vi "ContCompilePreSeq.vi"(11 "Compiler Settings In":T3={"Python Path"=path "", "Main File"="", "Meta File"="", "Aux File"="makesequence.py", "Pre File"="metascript.txt"}) -> (3 "Pre Pulse Seq":T1)   [LabVIEW 2019]
uses:
  PulseCompiler/CompilerSettings.ctl
  PulseControl.ctl
  Compiler/Params.ctl
panel:
  out "error out 2":errorcluster
  in  "Stepnum":i32
  out "standard error":string
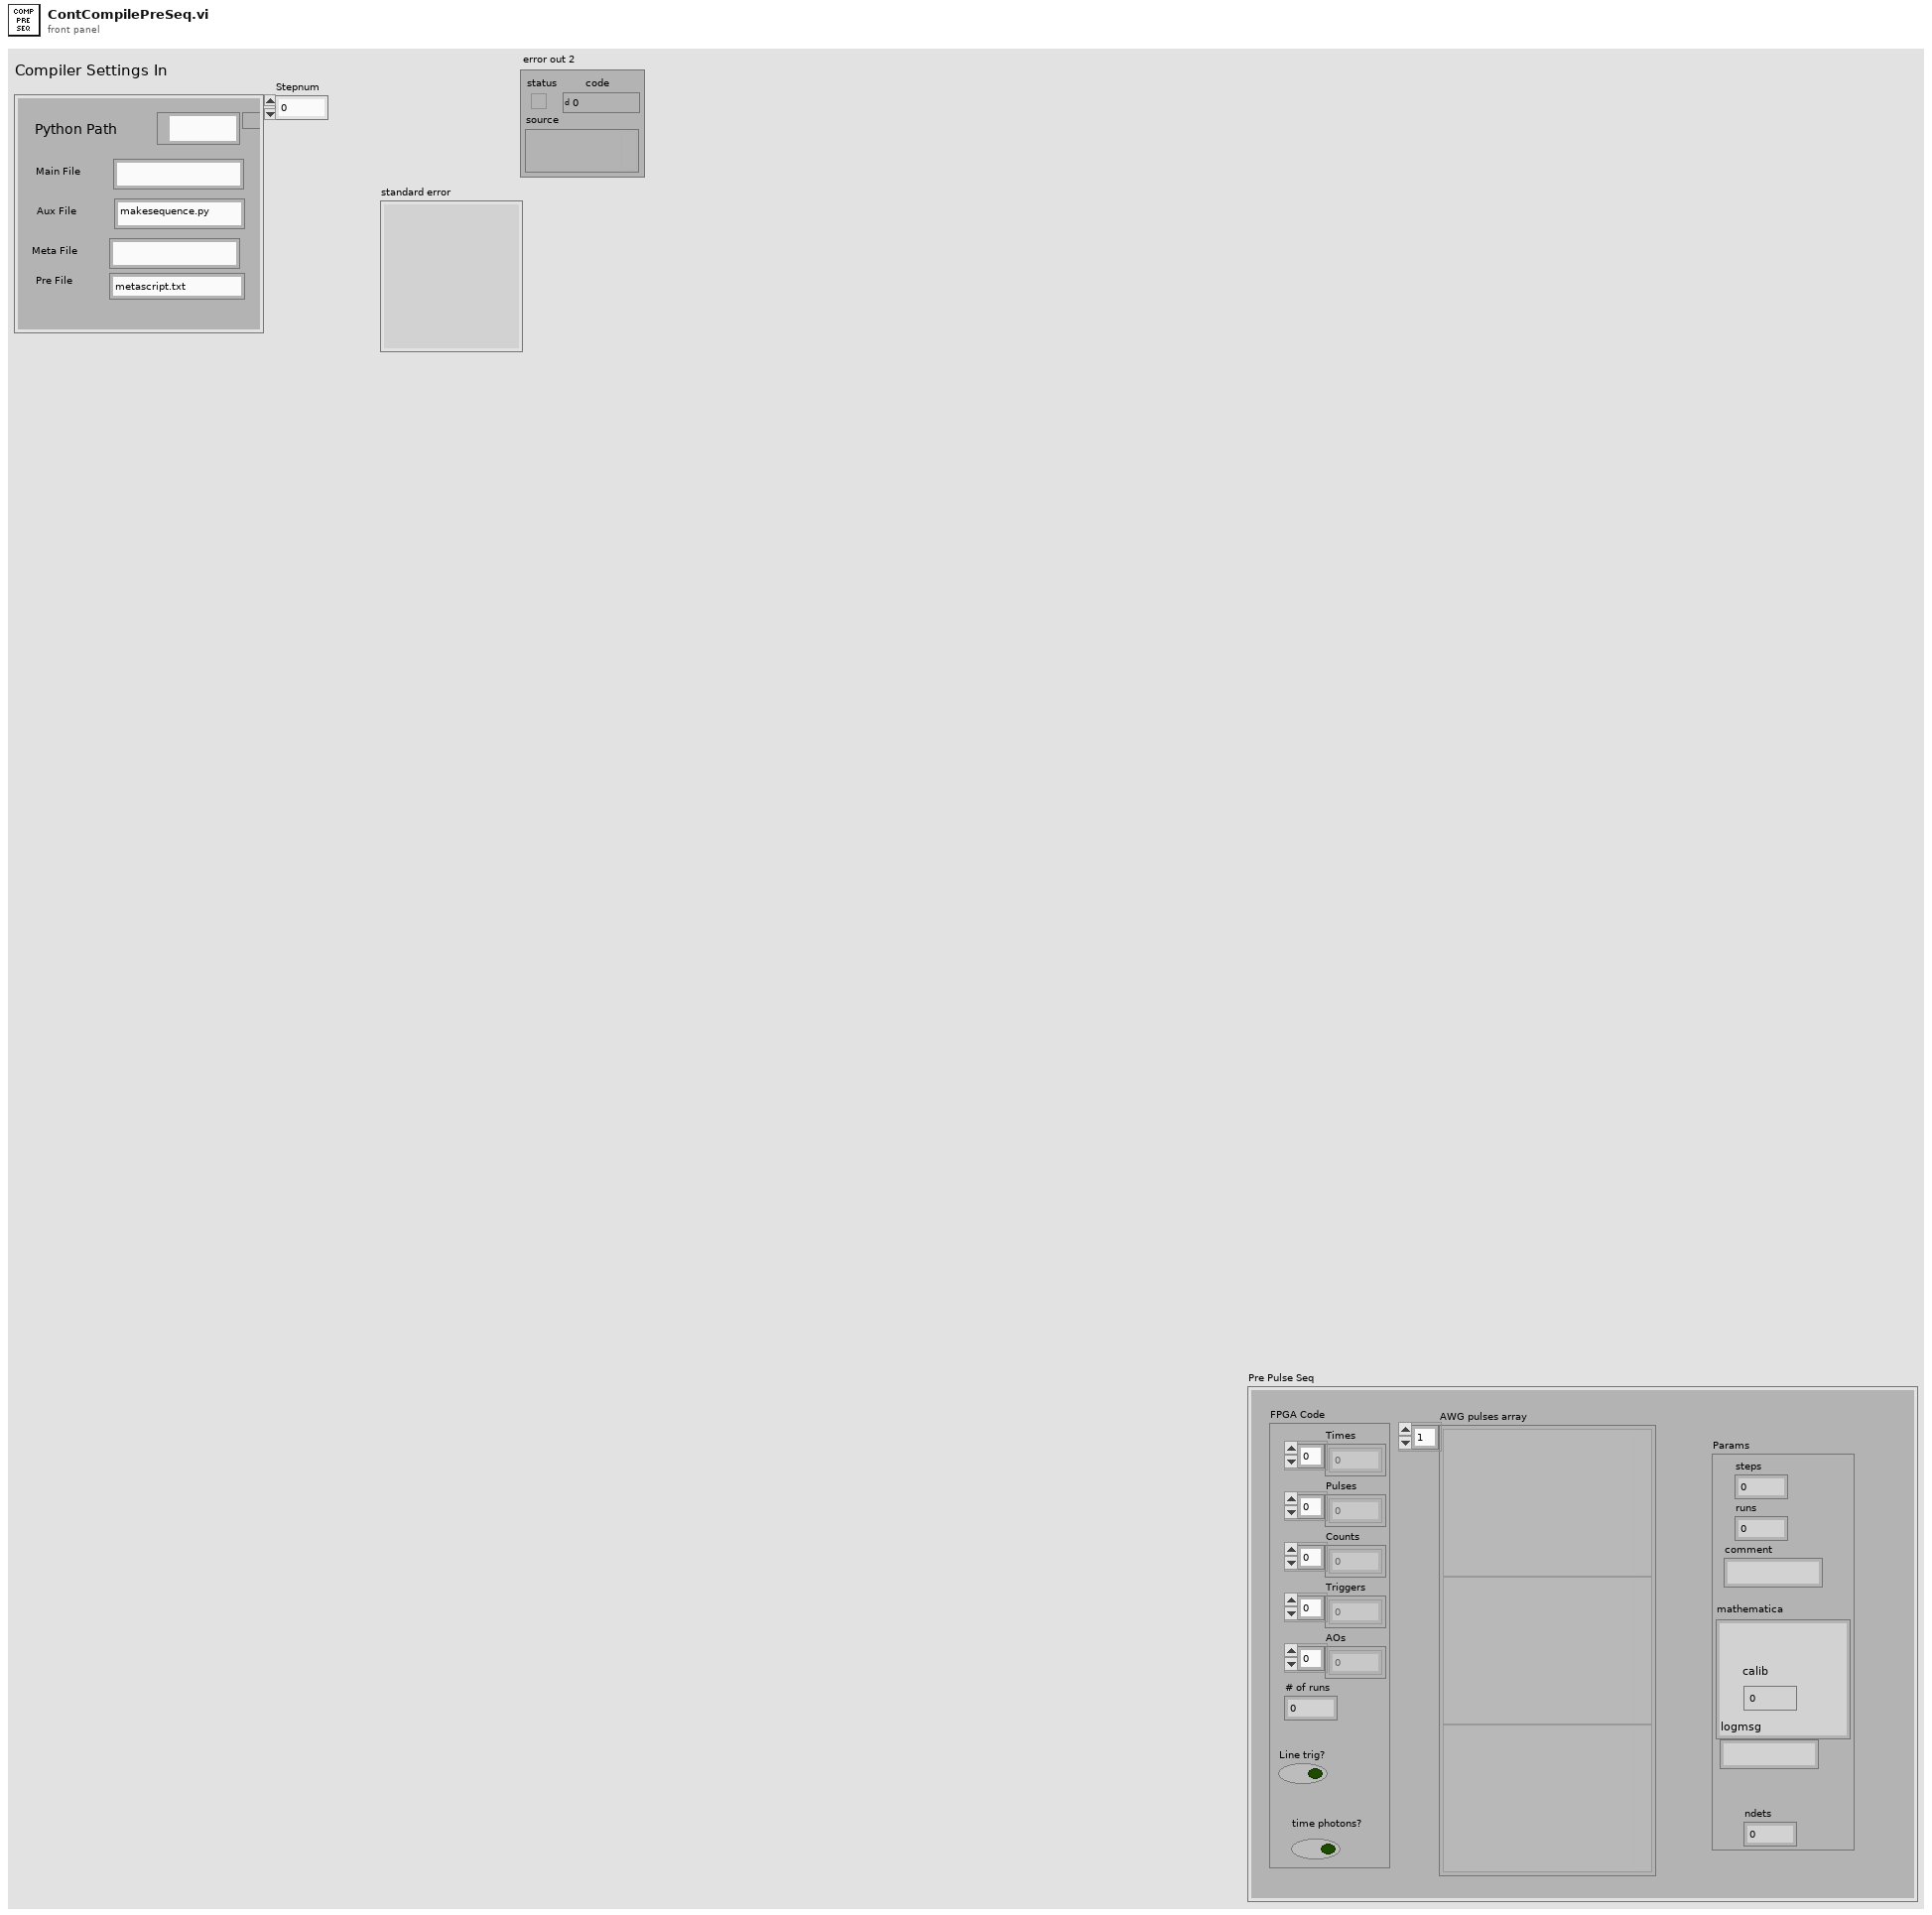
[diagram p1: front panel]
types:
  T1 = typedef "PulseControl.ctl" = cluster{"FPGA Code":cluster{"Times":u32[], "Pulses":u64[], "Counts":u8[], "Triggers":u8[], "AOs":u8[], "# of runs":i32, "Line trig?":bool, "time photons?":bool}, "AWG pulses array":variant[], "Params":T2}
  T2 = typedef "Params.ctl" = cluster{"steps":i16, "runs":i16, "comment":string, "mathematica":string, "calib":i8, "logmsg":string, "ndets":i16}
  T3 = typedef "CompilerSettings.ctl" = cluster{"Python Path":path, "Main File":string, "Meta File":string, "Aux File":string, "Pre File":string}
  T4 = typedef "SinglePulse.ctl" = cluster{"enabled":bool, "string":string, "time":dbl, "step":dbl, "dio":dbl, "count":dbl, "trigger":dbl, "AO":dbl}
  T5 = cluster{u32[], dbl[], "Count":dbl[], dbl[], dbl[], "# of runs":i32, "Line trig":bool, "save photon times":bool}
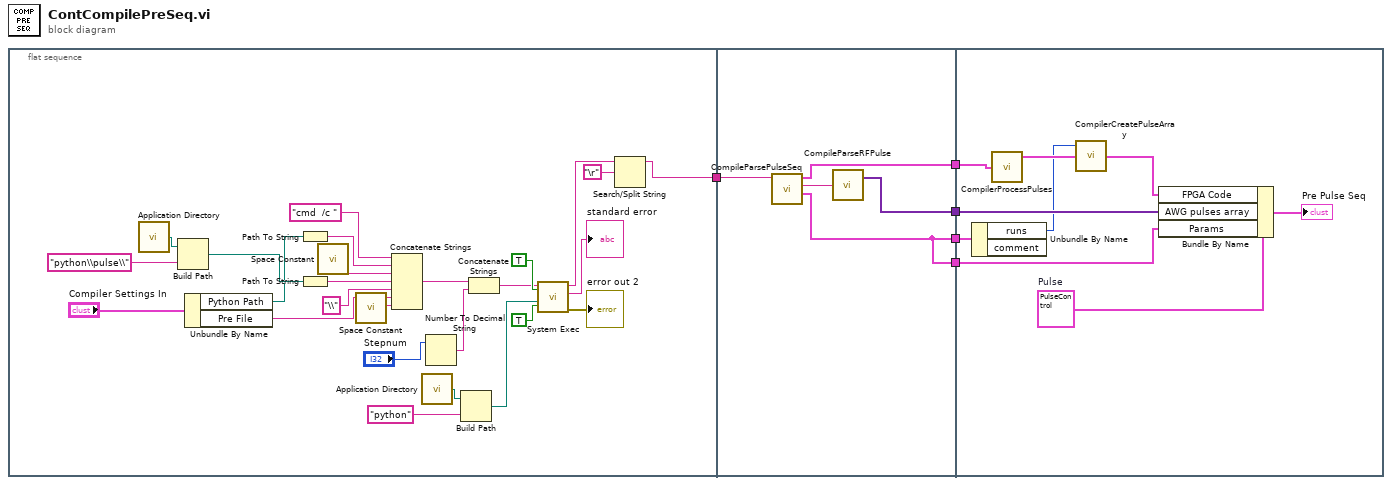
[diagram p0: block diagram]
diagram:
  n1 = flat-sequence {
    tunnel: [w6] -> w5
    tunnel: w5 -> [w35]
    tunnel: [w34] -> w4
    tunnel: [w33] -> w3
    tunnel: [w32] -> w2
    tunnel: [w32] -> w1
    tunnel: w4 -> [w45]
    tunnel: w3 -> [w41]
    tunnel: w2 -> [w40]
    tunnel: w1 -> [w38]
    frame #0 {
      n2 = call <vilib>:"Application Directory.vi"() -> ("Application Directory"=w24:path)
      n3 = Build Path(base path=w24, name or relative path="python\\pulse\\") -> (appended path=w26:path)
      n4 = Unbundle By Name("Compiler Settings In") -> ("Python Path"=w7:path, "Pre File"=w10:string)
      n5 = Path To String(path=w7) -> (string=w8:string)
      n6 = Path To String(path=w26) -> (string=w27:string)
      n7 = call <vilib>:"Space Constant.vi"() -> ("String"=w22:string)
      n8 = call <vilib>:"Space Constant.vi"() -> ("String"=w28:string)
      n9 = Concatenate Strings("cmd  /c " ("string"), w8, w22, w27, "\\" ("string"), w10, w28) -> (w23:string)
      n10 = call <vilib>:"Application Directory.vi"() -> ("Application Directory"=w16:path)
      n11 = Number To Decimal String(number="Stepnum") -> (decimal integer string=w14:string)  [unwired: 1 in]
      n12 = Build Path(base path=w16, name or relative path="python") -> (appended path=w18:path)
      n13 = Concatenate Strings(w23, w14) -> (w15:string)
      n14 = call <vilib>:"System Exec.vi"("run minimized? (F)"=TRUE, "wait until completion? (T)"=TRUE, "working directory"=w18, "command line"=w15) -> ("error out"=→"error out 2":errorcluster, "standard error"=→"standard error":string, "standard output"=w12:string)  [unwired: 4 in, 1 out]
      n15 = Search/Split String(string=w12, search string/char (-)="\r") -> (substring before match=w6:string)  [unwired: 1 in, 2 out]
    }
    frame #1 {
      n16 = call "CompileParsePulseSeq.vi"("PulseSeqIn"=w35) -> ("Params"=w32:T2, "RFPulseList"=w36:string, "PulseList"=w34:T4[])  [unwired: 7 in, 1 out]
      n17 = call "CompileParseRFPulse.vi"("String"=w36) -> ("Array"=w33:variant[])  [unwired: 1 in]
    }
    frame #2 {
      w43 = T1 {"FPGA Code"={"Times"=[], "Pulses"=[], "Counts"=[], "Triggers"=[], "AOs"=[], "# of runs"=0, "Line trig?"=FALSE, "time photons?"=FALSE}, "AWG pulses array"=[], "Params"={"steps"=0, "runs"=0, "comment"="", "mathematica"="", "calib"=0, "logmsg"="", "ndets"=0}}  # Pulse
      n18 = Unbundle By Name(w40) -> ("runs"=w39:i16)  [unwired: 1 out]
      n19 = call "CompilerProcessPulses.vi"("Pulse Seq In"=w45) -> ("Pulse Seq Out"=w44:T4[])  [unwired: 2 out]
      n20 = call "CompilerCreatePulseArray.vi"("Pulse Seq In"=w44, "runs"=w39) -> ("Pulse Seq Out"=w42:T5)  [unwired: 1 in]
      n21 = Bundle By Name(cluster=w43, "FPGA Code"=w42, "AWG pulses array"=w41, "Params"=w38) -> (→"Pre Pulse Seq":T1)
    }
  }
